vi "20-sub-2-Num to Array of Digits.vi"(3 "N":u64) -> (1 "N as Array of Digits":u8[](array[numeric]))   [LabVIEW 2021]
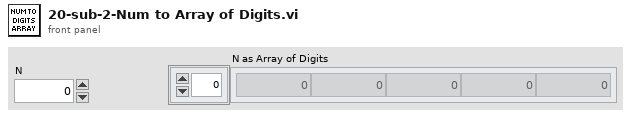
[diagram p1: front panel]
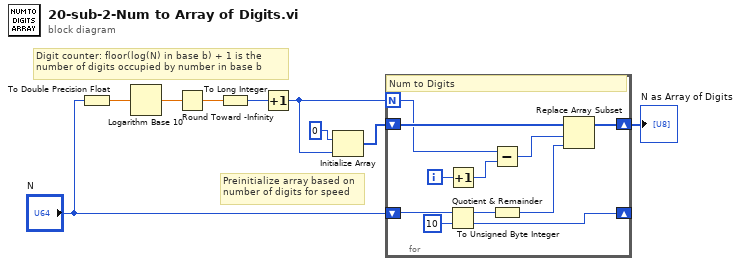
[diagram p0: block diagram]
diagram:
  # "Digit counter: floor(log(N) in base b) + 1 is the\nnumber of digits occupied by number in base b"
  # "Preinitialize array based on\nnumber of digits for speed"
  n1 = To Double Precision Float(number="N") -> (double precision float=w6:dbl)
  n2 = Logarithm Base 10(1:w6) -> (0:w9:dbl)
  n3 = Round Toward -Infinity(1:w9) -> (0:w8:dbl)
  n4 = To Long Integer(number=w8) -> (32bit integer=w7:i32)
  n5 = Increment(x=w7) -> (x+1=w2:i32)
  n6 = Initialize Array(u8 0, w2) -> (w3:u8[])
  n7 = for {
    N: w2 -> [w11]
    shift-right: [w18] -> _
    shift-left: "N" -> [w20]
    shift-right: [w16] -> w1
    shift-left: w3 -> [w17]
    i -> [w15]
    # "Num to Digits"
    n8 = Increment(x=w15) -> (x+1=w10:i32)
    n9 = Quotient & Remainder(x=w20, y=u64 10) -> (x-y*floor(x/y)=w14:u64, floor(x/y)=w18:u64)
    n10 = Subtract(x=w11, y=w10) -> (x-y=w12:i32)
    n11 = To Unsigned Byte Integer(number=w14) -> (unsigned 8bit integer=w13:u8)
    n12 = Replace Array Subset(array=w17, new element=w13, index=w12) -> (w16:u8[])
  }
  "N as Array of Digits" <- w1
